vi "Get User Attribute Value.vi"(0 "User Configuration Manager in":refnum<class "User Configuration Manager.lvclass">, 5 "Username":string, 7 "Attribute Name":string, 11 "error in (no error)":errorcluster) -> (4 "User Configuration Manager out":refnum<class "User Configuration Manager.lvclass">, 6 "Attribute Value":variant, 8 "Found":bool, 15 "error out":errorcluster)   [LabVIEW 2017, in "User Configuration Manager.lvlib" / "User Configuration Manager.lvclass"]
doc: "Gets the attribute's value specified by attribute name from the user specified by user name."
uses:
  User Configuration Manager.lvclass
  User Configuration Manager.lvclass/User Configuration Manager.ctl
  64f5a260-1ac1-421f-b717-63d5237117ec.vi
  Accessors/Read Linked List Ref .vi
  <vilib>/gpm_packages/@cs/linked-list/Source/Linked List/ILinkedList/ILinked List.lvclass
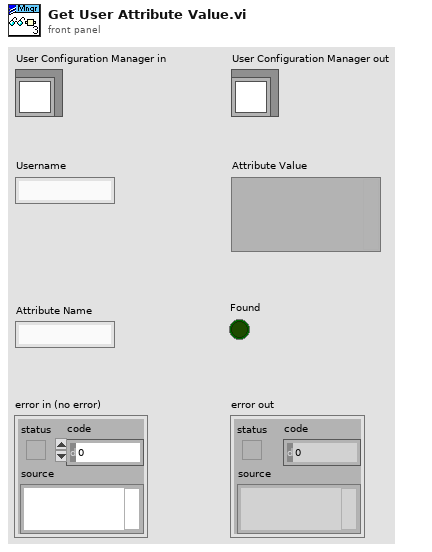
[diagram p1: front panel]
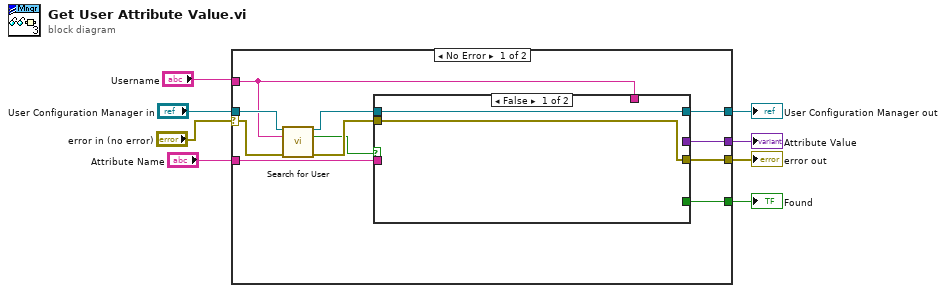
[diagram p0: block diagram]
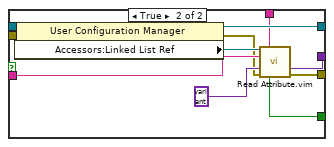
[diagram p2: hidden frame]
diagram:
  n1 = case shown="No Error" "error in (no error)" {
    selector: "error in (no error)" -> [w12 w33]
    tunnel: "User Configuration Manager in" -> [w14 w34]
    tunnel: "Attribute Name" -> [w16 _]
    tunnel: "Username" -> [w10 _]
    tunnel: [w19 w34] -> w4
    tunnel: [w18 _] -> w2
    tunnel: [w15 w33] -> w3
    tunnel: [w17 _] -> w1
    frame No Error {
      n2 = call-dynamic "Search for User.vi"("User Configuration Manager in"=w14, "Username"=w10, "error in (no error)"=w12) -> ("User Configuration Manager out"=w13:refnum<class "User Configuration Manager.lvclass">, "Found"=w9:bool, "error out"=w11:errorcluster)  [unwired: 10 in]
      n3 = case shown="False" w9 {
        tunnel: w13 -> [w21 w32]
        tunnel: [w21 w31] -> w19
        tunnel: w11 -> [w20 w30]
        tunnel: w10 -> [_ w28]
        tunnel: [_ w27] -> w18
        tunnel: [_ w26] -> w17
        tunnel: w16 -> [_ w25]
        tunnel: [w20 w22] -> w15
        frame False {
        }
        frame True {
          n4 = property class="User Configuration Manager"(reference=w32, error in=w30) -> (reference out=w31:refnum<class "User Configuration Manager.lvclass">, error out=w23:errorcluster, "Accessors:Linked List Ref "=w29:refnum<data-value>)
          n5 = call "Read Attribute.vim"("Linked List Ref"=w29, "Linked List ID"=w28, "Attribute Name"=w25, "Type"=variant, "error in (no error)"=w23) -> ("Attribute"=w27:variant, "Found?"=w26:bool, "error out"=w22:errorcluster)  [unwired: 5 in, 3 out]
        }
      }
    }
    frame Error {
    }
  }
  "error out" <- w3
  "User Configuration Manager out" <- w4
  "Attribute Value" <- w2
  "Found" <- w1
